vi "Command Translate Time Robot.vi"(2 "Input Robot System Funtions":T1, 3 "Cmd Parameter 1":dbl, 4 "Cmd Parameter 2":dbl, 5 "Startup":bool) -> (0 "Output Robot System Functions":T1, 1 "Completed":bool)   [LabVIEW 2014]
uses:
  Subsystems VIs/Robot Commands.ctl
  Command Execution State.ctl
panel:
  # "Sample robot\ncontrol output.\nReplace with \nactual teleop \ncontrol signal \nstructure."
  # "Field Centric"
  # "Field Centric"
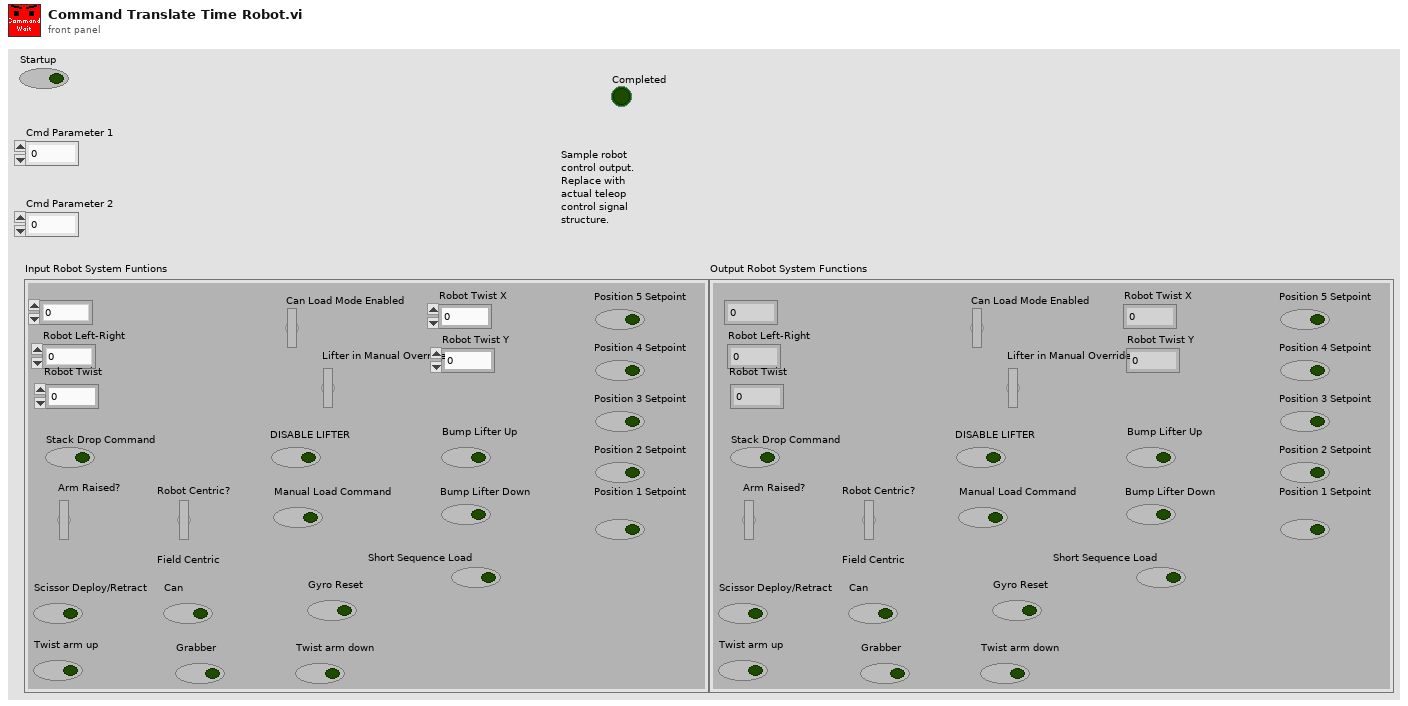
[diagram p1: front panel]
types:
  T1 = typedef "Robot Commands.ctl" = cluster{"Robot Forward-Reverse":dbl, "Robot Left-Right":dbl, "Robot Twist":dbl, "Can Load Mode Enabled":bool, "Lifter in Manual Override?":bool, "Stack Drop Command":bool, "Arm Raised?":bool, "DISABLE LIFTER":bool, "Position 1 Setpoint":bool, "Position 2 Setpoint":bool, "Position 3 Setpoint":bool, "Position 4 Setpoint":bool, "Position 5 Setpoint":bool, "Bump Lifter Down":bool, "Bump Lifter Up":bool, "Manual Load Command":bool, "Robot Centric?":bool, "Scissor Deploy/Retract":bool, "Grabber":bool, "Can":bool, "Twist arm up":bool, "Gyro Reset":bool, "Twist arm down":bool, "Short Sequence Load":bool, "Robot Twist X":dbl, "Robot Twist Y":dbl}
  T2 = typedef "Command Execution State.ctl" = enum16{"Initialize", "Execute", "Finish"}
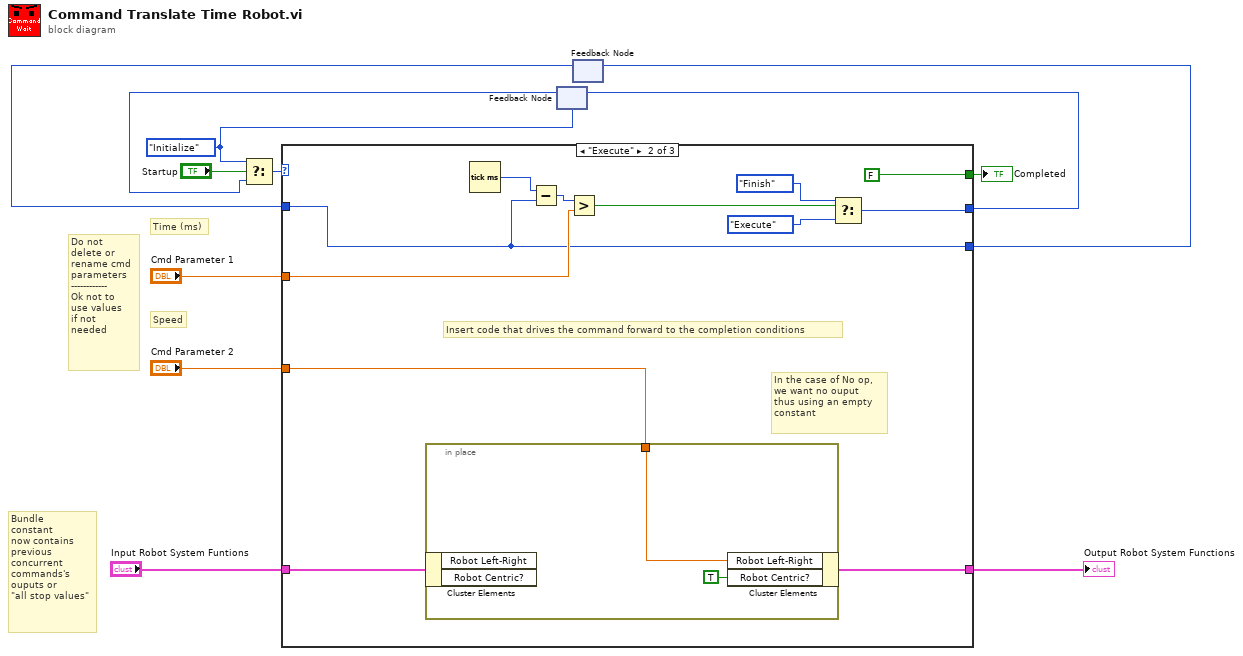
[diagram p0: block diagram]
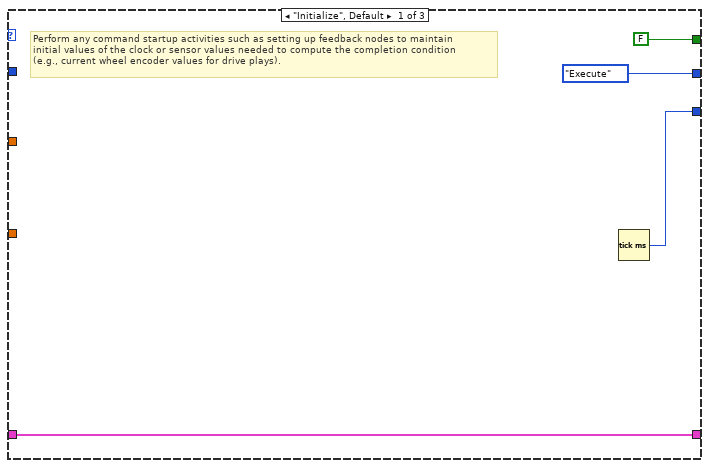
[diagram p2: hidden frame]
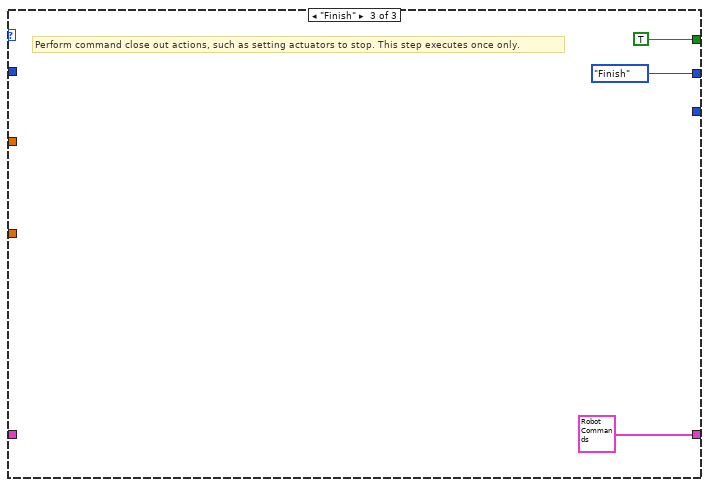
[diagram p3: hidden frame]
diagram:
  w7 = Command_Execution_State."Initialize" ("Play State")
  # "Bundle \nconstant\nnow contains\nprevious \nconcurrent\ncommands's\nouputs or\n\"all stop values\""
  # "Do not \ndelete or\nrename cmd\nparameters\n------------\nOk not to \nuse values\nif not \nneeded"
  # "Speed"
  # "Time (ms)"
  n1 = feedback #1(w7) -> (w8:T2)
  n2 = Select(t=w7, s="Startup", f=w8) -> (s? t:f=w12:T2)
  n3 = feedback #2() -> (w1:u32)  [unwired: 1 in]
  n4 = case shown="\"Execute\"" w12 {
    tunnel: [FALSE FALSE TRUE] -> w10
    tunnel: [Command_Execution_State."Execute" ("Play State") w19 Command_Execution_State."Finish" ("f")] -> w9
    tunnel: "Cmd Parameter 1" -> [_ w23 _]
    tunnel: "Cmd Parameter 2" -> [_ w26 _]
    tunnel: [w14 w27 T1 {"Robot Forward-Reverse"=0.0, "Robot Left-Right"=0.0, "Robot Twist"=0.0, "Can Load Mode Enabled"=FALSE, "Lifter in Manual Override?"=FALSE, "Stack Drop Command"=FALSE, "Arm Raised?"=FALSE, "DISABLE LIFTER"=FALSE, "Position 1 Setpoint"=FALSE, "Position 2 Setpoint"=FALSE, "Position 3 Setpoint"=FALSE, "Position 4 Setpoint"=FALSE, "Position 5 Setpoint"=FALSE, "Bump Lifter Down"=FALSE, "Bump Lifter Up"=FALSE, "Manual Load Command"=FALSE, "Robot Centric?"=FALSE, "Scissor Deploy/Retract"=FALSE, "Grabber"=FALSE, "Can"=FALSE, "Twist arm up"=FALSE, "Gyro Reset"=FALSE, "Twist arm down"=FALSE, "Short Sequence Load"=FALSE, "Robot Twist X"=0.0, "Robot Twist Y"=0.0} ("Input Robot System Funtions")] -> w3
    tunnel: "Input Robot System Funtions" -> [w14 w28 _]
    tunnel: w1 -> [_ w17 _]
    tunnel: [w13 w17 _] -> w2
    frame "Initialize", Default {
      # "Perform any command startup activities such as setting up feedback nodes to maintain \ninitial values of the clock or sensor values needed to compute the completion condition\n(e.g., current wheel encoder values for drive plays)."
      n5 = Tick Count (ms)() -> (millisecond timer value=w13:u32)
    }
    frame "Execute" {
      # "In the case of No op, \nwe want no ouput \nthus using an empty \nconstant"
      # "Insert code that drives the command forward to the completion conditions"
      n6 = in-place {
        in-place-border: w26 -> [w30]
        n7 = in-place-cluster #3(w28) -> ()  [unwired: 2 out]
        n8 = in-place-cluster #3("Robot Left-Right"=w30, "Robot Centric?"=TRUE) -> (w27:T1)
      }
      n9 = Tick Count (ms)() -> (millisecond timer value=w25:u32)
      n10 = Subtract(x=w25, y=w17) -> (x-y=w24:u32)
      n11 = Greater?(x=w24, y=w23) -> (0:w21:bool)
      n12 = Select(t=Command_Execution_State."Finish" ("Play State"), s=w21, f=Command_Execution_State."Execute" ("Play State")) -> (s? t:f=w19:T2)
    }
    frame "Finish" {
      # "Perform command close out actions, such as setting actuators to stop. This step executes once only."
    }
  }
  "Completed" <- w10
  "Output Robot System Functions" <- w3
  n13 = feedback-in #1(w9) -> ()
  n14 = feedback-in #2(w2) -> ()
